vi "load_cell_mea.vi"() -> ()   [LabVIEW 2024]
uses:
  <vilib>/xnet/xnet.llb/XNET Create Session (Signal Input Single-point).vi
  <vilib>/xnet/xnet.llb/XNET Read (Signal Single-point).vi
  <resource>/objmgr/xnet.rc
panel:
  out "Waveform Chart 2":cluster{dbl, dbl}(graph)
  out "1/x":dbl
  out "Waveform Chart":cluster{dbl, dbl, dbl, dbl}(graph)
  in  "stop":bool
  out "data":dbl[](array[numeric]) format="%.2f"
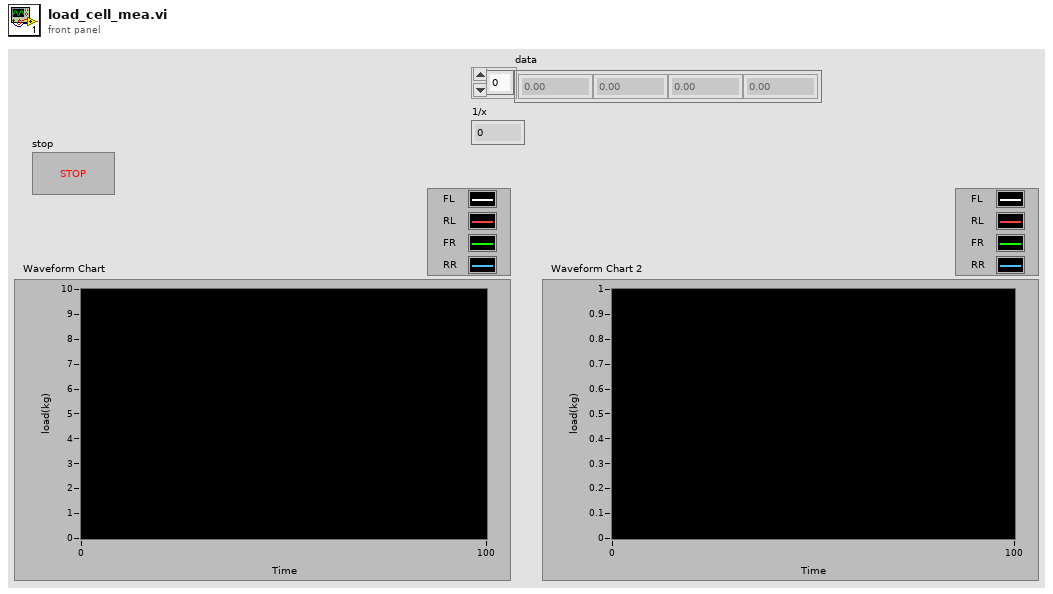
[diagram p1: front panel]
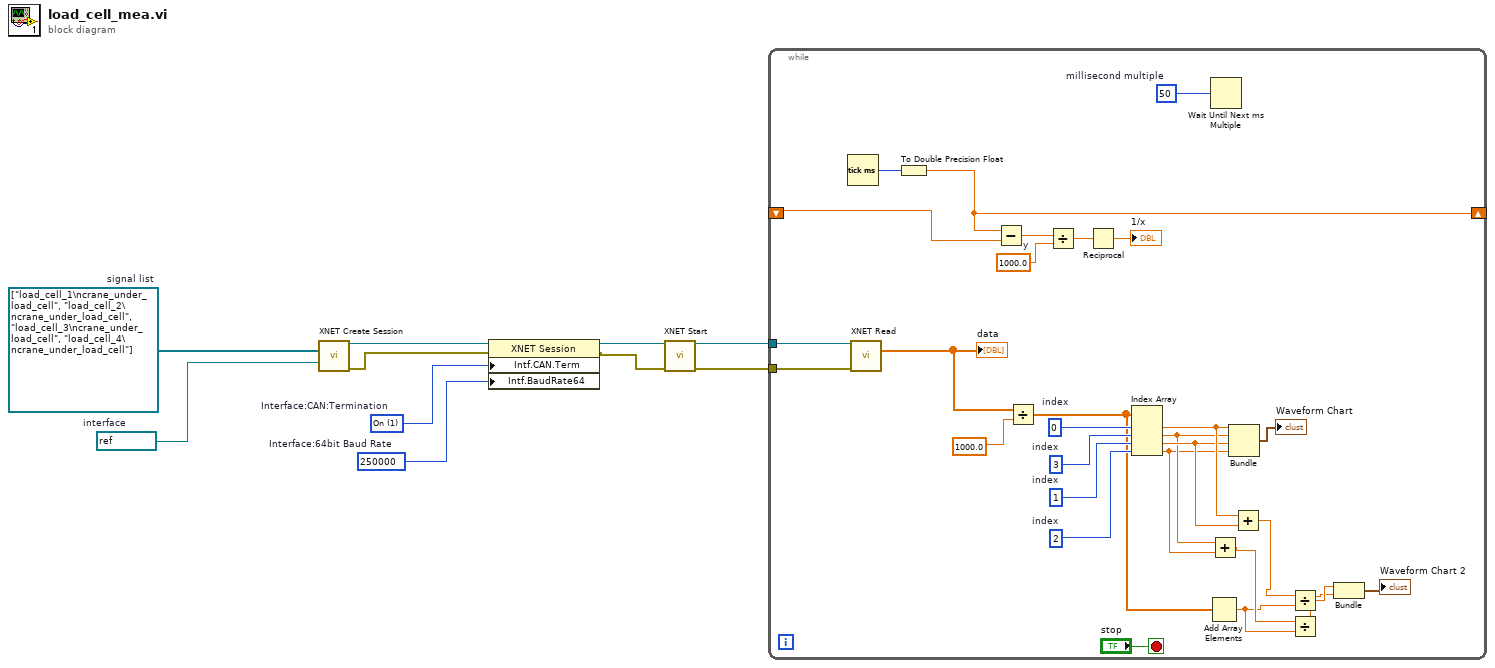
[diagram p0: block diagram]
diagram:
  w5 = u64 250000  # Interface:64bit Baud Rate
  w6 = u32 1 items=["Off", "On"]  # Interface:CAN:Termination
  w8 = refnum<k21> "CAN1"  # interface
  w10 = refnum<k21>[] ["load_cell_1\ncrane_under_load_cell", "load_cell_2\ncrane_under_load_cell", "load_cell_3\ncrane_under_load_cell", "load_cell_4\ncrane_under_load_cell"]  # signal list
  n1 = call-poly <vilib>:"XNET Create Session.vi"("signal list"=w10, "interface"=w8) -> ("session out"=w9:refnum<k21>, "error out"=w7:errorcluster)  [unwired: 12 in]
  n2 = property class="XNET Session"(reference=w9, error in=w7, "Intf.CAN.Term"=w6, "Intf.BaudRate64"=w5) -> (reference out=w4:refnum<k21>, error out=w3:errorcluster)
  n3 = call <vilib>:"XNET Start.vi"("session in"=w4, "error in (no error)"=w3) -> ("session out"=w2:refnum<k21>, "error out"=w1:errorcluster)  [unwired: 12 in]
  n4 = while {
    tunnel: w2 -> [w39]
    tunnel: w1 -> [w38]
    shift-right: [w35] -> _
    shift-left: _ -> [w34]
    stop <- "stop" stop-if-true
    w23 = 2  # index
    w24 = 1  # index
    w25 = 3  # index
    w26 = 0  # index
    w29 = u32 50  # millisecond multiple
    w32 = 1000.0  # y
    n5 = Tick Count (ms)() -> (millisecond timer value=w36:u32)
    n6 = call-poly <vilib>:"XNET Read.vi"("session in"=w39, "error in (no error)"=w38) -> ("data"=w28:dbl[])  [unwired: 11 in, 2 out]
    "data" <- w28
    n7 = To Double Precision Float(number=w36) -> (double precision float=w35:dbl)
    n8 = Subtract(x=w35, y=w34) -> (x-y=w33:dbl)
    n9 = Divide(x=w28, y=1000.0) -> (x/y=w17:dbl[])
    n10 = Divide(x=w33, y=w32) -> (x/y=w31:dbl)
    n11 = Reciprocal(x=w31) -> (1/x=→"1/x":dbl)
    n12 = Index Array(array=w17, index #1=w26, index #2=w25, index #3=w24, index #4=w23) -> (element #1=w21:dbl, element #2=w19:dbl, element #3=w20:dbl, element #4=w18:dbl)
    n13 = Add Array Elements(numeric array=w17) -> (sum=w14:dbl)
    n14 = Add(x=w19, y=w18) -> (x+y=w15:dbl)
    n15 = Wait Until Next ms Multiple(millisecond multiple=w29) -> ()  [unwired: 1 out]
    n16 = Bundle(w21, w19, w20, w18) -> (→"Waveform Chart":cluster{dbl, dbl, dbl, dbl})  [unwired: 1 in]
    n17 = Add(x=w21, y=w20) -> (x+y=w16:dbl)
    n18 = Divide(x=w16, y=w14) -> (x/y=w13:dbl)
    n19 = Divide(x=w15, y=w14) -> (x/y=w12:dbl)
    n20 = Bundle(w13, w12) -> (→"Waveform Chart 2":cluster{dbl, dbl})  [unwired: 1 in]
  }
